vi "DB Tools Set Properties.vi"   [LabVIEW 2020, in "NI_Database_API.lvlib"]
doc: "Sets properties on the object as determined by the inputs. Wire data to the reference and properties inputs to determine the polymorphic instance to use or manually select the instance."
uses:
  <vilib>/addons/database/NI_Database_API.lvlib
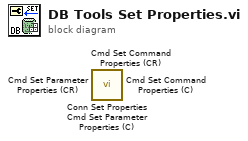
[diagram p0: block diagram]
diagram:
  n1 = call <vilib>:"Conn Set Properties.vi"() -> ()  [unwired: 6 in, 2 out]
  n2 = call <vilib>:"Cmd Set Command Properties (CR).vi"() -> ()  [unwired: 6 in, 2 out]
  n3 = call <vilib>:"Cmd Set Parameter Properties (CR).vi"() -> ()  [unwired: 6 in, 2 out]
  n4 = call <vilib>:"Cmd Set Command Properties (C).vi"() -> ()  [unwired: 6 in, 2 out]
  n5 = call <vilib>:"Cmd Set Parameter Properties (C).vi"() -> ()  [unwired: 6 in, 2 out]
